vi "EvaluateOpStateExit.vi"(8 "error in (no error)":errorcluster, 9 "data flow":T2, 10 "config":T1, 11 "Qbus":refnum<class "Qbus.lvclass">) -> (0 "error out":errorcluster, 2 "config out":T1)   [LabVIEW 2017, in "CmsDataEventCreator.lvlib"]
uses:
  <vilib>/addons/InsightCM/Devices/Shared/Cms/CmsDataEventCreator/CmsDataEventCreator.lvlib
  <vilib>/addons/InsightCM/Devices/Shared/Common/DataFlow/controls/Data.ctl
  <vilib>/addons/InsightCM/Utilities/DataAccessors/controls/wfmSGL_DVR.ctl
  <vilib>/addons/PointValueMap/controls/PointMap.ctl
  <vilib>/addons/InsightCM/Devices/Shared/Common/DataFlow/controls/Type.ctl
  <vilib>/addons/Qbus/Qbus.lvclass
  <vilib>/addons/InsightCM/Devices/Shared/Cms/CmsDataEventCreator/controls/config.ctl
  <vilib>/addons/InsightCM/Devices/Shared/Cms/CmsDataEventCreator/controls/AcqParams.ctl
  <vilib>/addons/InsightCM/Devices/Shared/Common/DataAccumulator/controls/AccumulationSettings.ctl
  <vilib>/addons/InsightCM/Devices/Shared/Common/DataAccumulator/controls/accumulationType.ctl
  <vilib>/addons/InsightCM/Devices/Shared/Common/DVRBuffer/controls/BufferLocation.ctl
  <vilib>/addons/InsightCM/MessageBus/MessageLibrary/DataStorage/controls/DataStorageCloseStreamRoutedMessageBody.ctl
  <vilib>/addons/InsightCM/Devices/Shared/Cms/CmsDataEventCreator/controls/DataEventConfig.ctl
  <vilib>/addons/InsightCM/Devices/Shared/Common/DataEventCreator/controls/Reason.ctl
  <vilib>/addons/PointValueMap/subVIs/Point_Read_string.vi
  <vilib>/addons/PointValueMap/PointValueMap.lvlib
  <vilib>/addons/InsightCM/Devices/Shared/Common/DataEventCreator/DataEventCreator.lvlib
  <vilib>/addons/InsightCM/Devices/Shared/Common/DVRBuffer/DVRBuffer.lvlib
  <vilib>/addons/InsightCM/Devices/Shared/Common/DataAccumulator/DataAccumulator.lvlib
  <vilib>/addons/InsightCM/Devices/Shared/Common/DataFlow/DataFlow.lvlib
  <vilib>/addons/InsightCM/Devices/Shared/Common/ServerComm/ServerComm.lvlib
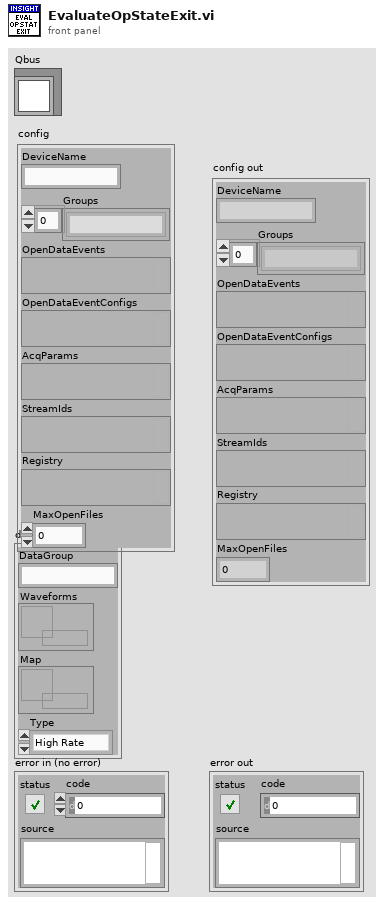
[diagram p1: front panel]
types:
  T1 = typedef "CmsDataEventCreator.lvlib/config.ctl" = cluster{"DeviceName":string, "Groups":string[], "OpenDataEvents":variant, "OpenDataEventConfigs":variant, "AcqParams":variant, "StreamIds":variant, "Registry":variant, "MaxOpenFiles":i32}
  T2 = typedef "DataFlow.lvlib/Data.ctl" = cluster{"DataGroup":string, "Waveforms":T3, "Map":T4, "Type":T5}
  T3 = typedef "wfmSGL_DVR.ctl" = refnum<data-value>
  T4 = typedef "PointValueMap.lvlib/PointMap.ctl" = refnum<data-value>
  T5 = typedef "DataFlow.lvlib/Type.ctl" = enum16{"High Rate", "Low Rate", "Burst Mode"}
  T6 = typedef "CmsDataEventCreator.lvlib/AcqParams.ctl" = cluster{"Stream":bool, "PreTrigger":i32, "CollectOnEnter":bool, "Enter PreTrigger":i32, "Enter Length":dbl, "CollectOnExit":bool, "ContinuousData":bool, "Accumulation Settings":T7}
  T7 = typedef "DataAccumulator.lvlib/AccumulationSettings.ctl" = cluster{"Type":T8, "Length":dbl, "Max Time (sec)":dbl, "Start Block":T9, "Acquired (sec)":dbl, "Acquired (pulses)":i32, "Initial Pulse Offset":dbl, "Stop Block":T9, "LastBlockAdded":u32}
  T8 = typedef "DataAccumulator.lvlib/accumulationType.ctl" = enum16{"none", "seconds", "revolutions"}
  T9 = typedef "DVRBuffer.lvlib/BufferLocation.ctl" = cluster{"Block":u32, "Index":i32}
  T10 = typedef "DataStorageCloseStreamRoutedMessageBody.ctl" = cluster{"StreamId":string}
  T11 = typedef "DataEventCreator.lvlib/Reason.ctl" = enum16{"Periodic Event", "Delta EU Event", "Trend Event", "Alarm Event", "User Event", "Enter Operating State", "Exit Operating State", "Multiple Events", "Other"}
  T12 = typedef "Message.ctl" = cluster{"Header":T13, "Body":u8[]}
  T13 = typedef "MessageHeader.ctl" = cluster{"MessageName":string, "Timestamp":i64, "CorrelationId":string, "ContentType":string, "RoutingKey":string, "Properties":T14[]}
  T14 = typedef "KeyValuePair.ctl" = cluster{"Key":string, "Value":string}
  T15 = typedef "CmsDataEventCreator.lvlib/DataEventConfig.ctl" = cluster{"AcqParams":T6, "OpState":string, "ExitOpState":bool, "Reason":string, "StreamId":string, "Map":T4, "DataSetIds":variant, "IncludeWaveforms":bool, "TrendPointsOnly":bool}
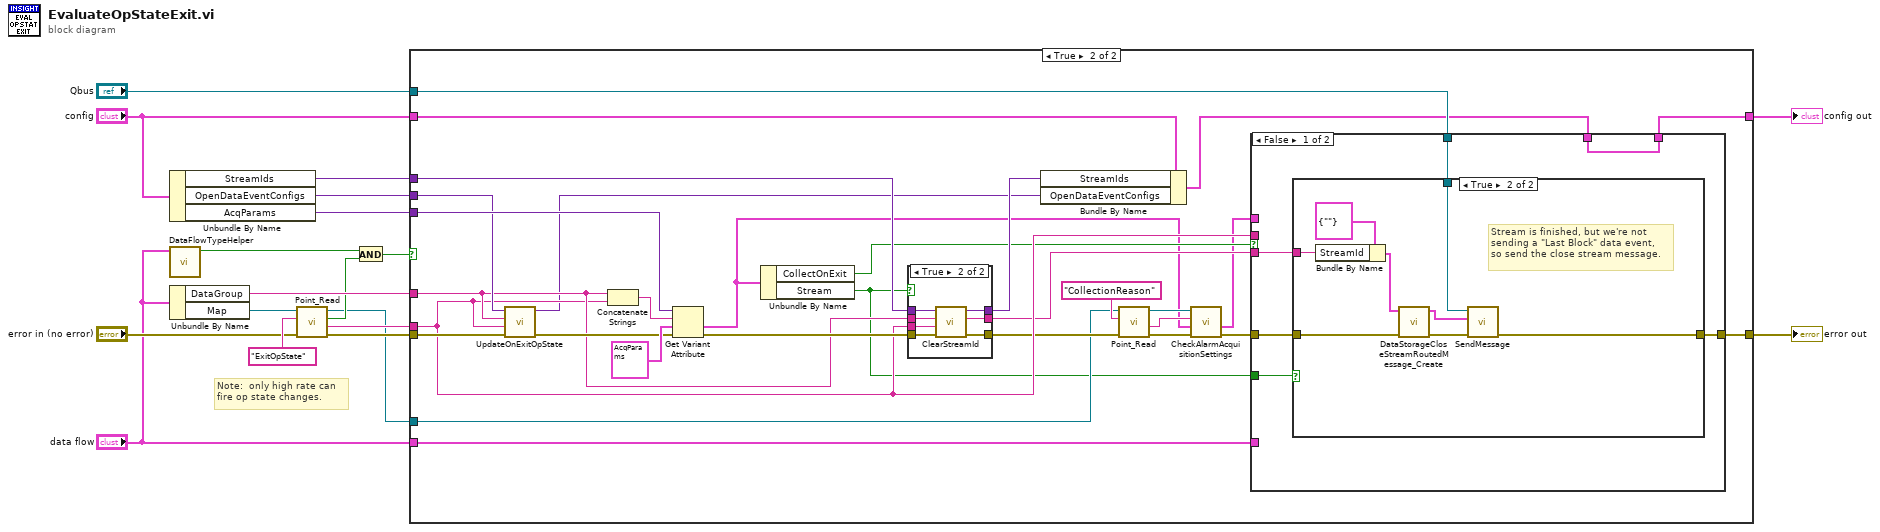
[diagram p0: block diagram]
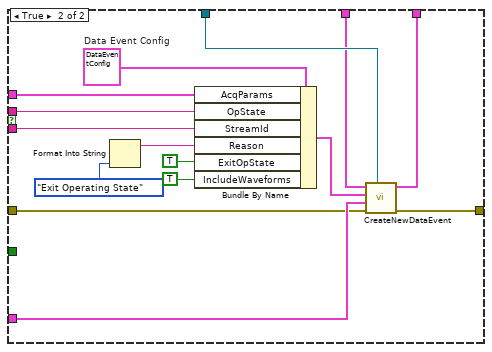
[diagram p4: hidden frame]
diagram:
  # "Note:  only high rate can\nfire op state changes."
  n1 = Unbundle By Name("config") -> ("StreamIds"=w12:variant, "OpenDataEventConfigs"=w8:variant, "AcqParams"=w7:variant)
  n2 = call <vilib>:"DataFlowTypeHelper.vi"("data"="data flow") -> ("high rate"=w1:bool)  [unwired: 8 in, 2 out]
  n3 = Unbundle By Name("data flow") -> ("DataGroup"=w13:string, "Map"=w18:T4)
  n4 = call-poly <vilib>:"Point_Read.vi"("Error In"="error in (no error)", "Tag"="ExitOpState", "Map"=w18) -> ("Error Out"=w15:errorcluster, "Value"=w14:string, "Found?"=w5:bool, "Map Out"=w3:T4)  [unwired: 3 in, 2 out]
  n5 = And(x=w1, y=w5) -> (x .and. y?=w4:bool)
  n6 = case shown="True" w4 {
    tunnel: w15 -> [w19 w38]
    tunnel: w14 -> [_ w34]
    tunnel: w13 -> [_ w35]
    tunnel: w7 -> [_ w49]
    tunnel: w12 -> [_ w46]
    tunnel: "config" -> [w20 w45]
    tunnel: [w20 w44] -> w10
    tunnel: "data flow" -> [_ w43]
    tunnel: "Qbus" -> [_ w42]
    tunnel: [w19 w41] -> w9
    tunnel: w8 -> [_ w36]
    tunnel: w3 -> [_ w24]
    frame False {
    }
    frame True {
      n7 = call <vilib>:"UpdateOnExitOpState.vi"("error in (no error)"=w38, "operating state"=w34, "data group"=w35, "open data event configs in"=w36) -> ("error out"=w37:errorcluster, "open data event configs out"=w33:variant)  [unwired: 6 in]
      n8 = Concatenate Strings(w35, w34) -> (w50:string)
      n9 = Get Variant Attribute(Variant=w49, name=w50, default value (empty Variant)=T6 {"Stream"=FALSE, "PreTrigger"=0, "CollectOnEnter"=FALSE, "Enter PreTrigger"=0, "Enter Length"=0.0, "CollectOnExit"=FALSE, "ContinuousData"=FALSE, "Accumulation Settings"={"Type"=enum."none", "Length"=0.0, "Max Time (sec)"=0.0, "Start Block"={"Block"=0, "Index"=0}, "Acquired (sec)"=0.0, "Acquired (pulses)"=0, "Initial Pulse Offset"=0.0, "Stop Block"={"Block"=0, "Index"=0}, "LastBlockAdded"=0}} ("AcqParams"), error in=w37) -> (value=w23:T6, error out=w47:errorcluster)  [unwired: 2 out]
      n10 = Unbundle By Name(w23) -> ("CollectOnExit"=w31:bool, "Stream"=w21:bool)
      n11 = case shown="True" w21 {
        tunnel: w47 -> [w81 w89]
        tunnel: w46 -> [w82 w88]
        tunnel: w35 -> [_ w87]
        tunnel: w34 -> [_ w86]
        tunnel: [w82 w85] -> w40
        tunnel: [_ w84] -> w32
        tunnel: [w81 w83] -> w26
        frame False {
        }
        frame True {
          n12 = call <vilib>:"ClearStreamId.vi"("error in (no error)"=w89, "operating state"=w86, "data group"=w87, "OpStateCorrIds in"=w88) -> ("error out"=w83:errorcluster, "operating state corrId"=w84:string, "OpStateCorrIds out"=w85:variant)  [unwired: 5 in]
        }
      }
      n13 = Bundle By Name(cluster=w45, "StreamIds"=w40, "OpenDataEventConfigs"=w33) -> (w39:T1)
      n14 = call-poly <vilib>:"Point_Read.vi"("Error In"=w26, "Tag"="CollectionReason", "Map"=w24) -> ("Error Out"=w29:errorcluster, "Value"=w28:string, "Map Out"=w27:T4)  [unwired: 3 in, 3 out]
      n15 = call <vilib>:"CheckAlarmAcquisitionSettings.vi"("error in (no error)"=w29, "acq config in"=w23, "collection reason"=w28, "map"=w27) -> ("error out"=w25:errorcluster, "acq config out"=w22:T6)  [unwired: 6 in]
      n16 = case shown="False" w31 {
        tunnel: w22 -> [_ w80]
        tunnel: [w56 w79] -> w44
        tunnel: w43 -> [_ w78]
        tunnel: w42 -> [w51 w77]
        tunnel: [w55 w76] -> w41
        tunnel: w25 -> [w54 w75]
        tunnel: w39 -> [w56 w74]
        tunnel: w34 -> [_ w73]
        tunnel: w32 -> [w52 w66]
        tunnel: w21 -> [w53 _]
        frame False {
          n17 = case shown="True" w53 {
            tunnel: [w57 w60] -> w55
            tunnel: w54 -> [w57 w61]
            tunnel: w52 -> [_ w59]
            tunnel: w51 -> [_ w58]
            frame False {
            }
            frame True {
              # "Stream is finished, but we're not\nsending a \"Last Block\" data event,\nso send the close stream message."
              n18 = Bundle By Name(cluster=T10 {"StreamId"=""} ("DataStorageCloseStreamRoutedMessage"), "StreamId"=w59) -> (w62:T10)
              n19 = call <vilib>:"DataStorageCloseStreamRoutedMessage_Create.vi"("error in (no error)"=w61, "DataStorageCloseStreamRoutedMessage"=w62) -> ("error out"=w64:errorcluster, "Message"=w65:T12)  [unwired: 8 in]
              n20 = call <vilib>:"SendMessage.vi"("error in (no error)"=w64, "message"=w65, "Qbus in"=w58) -> ("error out"=w60:errorcluster)  [unwired: 7 in, 1 out]
            }
          }
        }
        frame True {
          w72 = T15 {"AcqParams"={"Stream"=FALSE, "PreTrigger"=0, "CollectOnEnter"=FALSE, "Enter PreTrigger"=0, "Enter Length"=0.0, "CollectOnExit"=FALSE, "ContinuousData"=FALSE, "Accumulation Settings"={"Type"=enum."none", "Length"=0.0, "Max Time (sec)"=0.0, "Start Block"={"Block"=0, "Index"=0}, "Acquired (sec)"=0.0, "Acquired (pulses)"=0, "Initial Pulse Offset"=0.0, "Stop Block"={"Block"=0, "Index"=0}, "LastBlockAdded"=0}}, "OpState"="", "ExitOpState"=FALSE, "Reason"="", "StreamId"="", "Map"=refnum, "DataSetIds"=variant, "IncludeWaveforms"=FALSE, "TrendPointsOnly"=FALSE}  # Data Event Config
          n21 = Format Into String(Reason."Exit Operating State" ("Reason")) -> (resulting string=w67:string)  [unwired: 3 in, 1 out]
          n22 = Bundle By Name(cluster=w72, "AcqParams"=w80, "OpState"=w73, "StreamId"=w66, "Reason"=w67, "ExitOpState"=TRUE, "IncludeWaveforms"=TRUE) -> (w71:T15)
          n23 = call <vilib>:"CreateNewDataEvent.vi"("Qbus"=w77, "error in (no error)"=w75, "data flow"=w78, "data event config"=w71, "config"=w74) -> ("error out"=w76:errorcluster, "config out"=w79:T1)  [unwired: 5 in]
        }
      }
    }
  }
  "error out" <- w9
  "config out" <- w10
